vi "DVR To Obj.vi"(3 "RefIn":u32) -> (0 "error_out":errorcluster, 1 "data":refnum<class "SV Sinusoid.lvclass">)   [LabVIEW 2021]
uses:
  <vilib>/addons/_NISVFA/_Generation/Signal Generation/SV Sinusoid/SV Sinusoid.lvclass
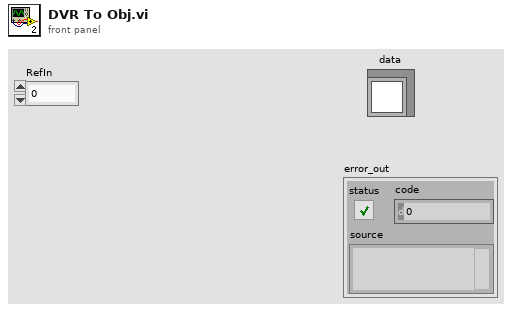
[diagram p1: front panel]
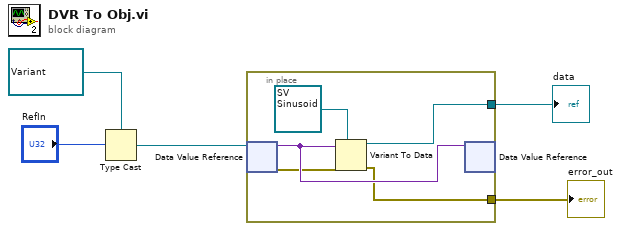
[diagram p0: block diagram]
diagram:
  n1 = Type Cast(type=refnum<data-value> refnum ("data value reference"), x="RefIn") -> (*(type *) &x=w3:refnum<data-value>)
  n2 = in-place {
    in-place-border: [w8] -> w2
    in-place-border: [w6] -> w1
    n3 = in-place-dvr #1(w3) -> (w10:variant, w9:errorcluster)
    n4 = Variant To Data(error in=w9, type=refnum<class "SV Sinusoid.lvclass"> refnum ("signal configuration"), Variant=w10) -> (data=w6:refnum<class "SV Sinusoid.lvclass">, error out=w8:errorcluster)
    n5 = in-place-dvr #1(w10) -> ()  [unwired: 2 out]
  }
  "error_out" <- w2
  "data" <- w1
